vi "Execute_Arc.vi"(2 "Type":u8(slide)=1 min=1 max=12 step=1 scale=1.0..12.0, 3 "Radius":i16 min=0, 4 "occurrence":refnum<k4>, 5 "Motor GPIB":u8=6) -> ()   [LabVIEW 2012]
uses:
  X-Y Go(Global).vi
  <vilib>/express/express arith-compare/Formula/XNode/ExpressFormulaBlockNode.xnode
panel:
  out "move x":i16
  out "move y":i16
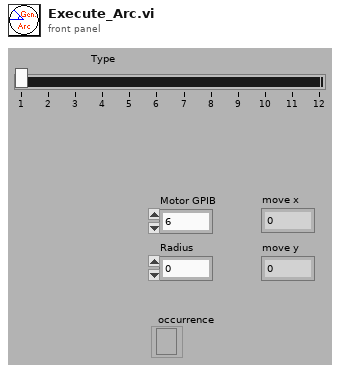
[diagram p1: front panel]
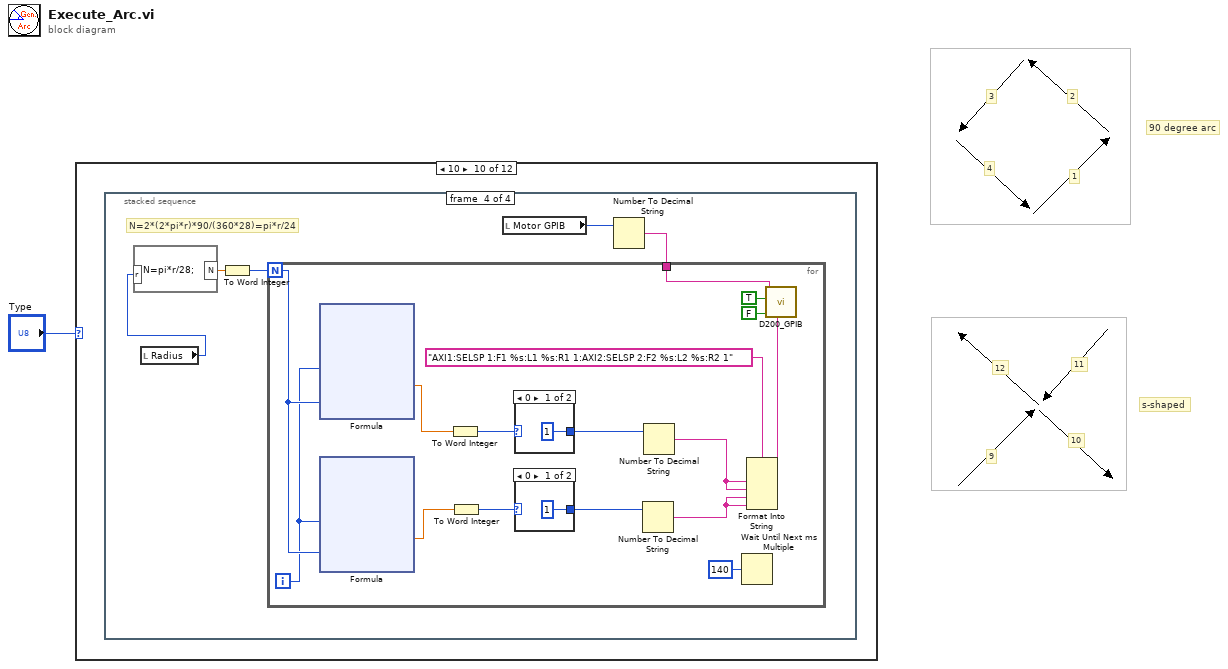
[diagram p0: block diagram]
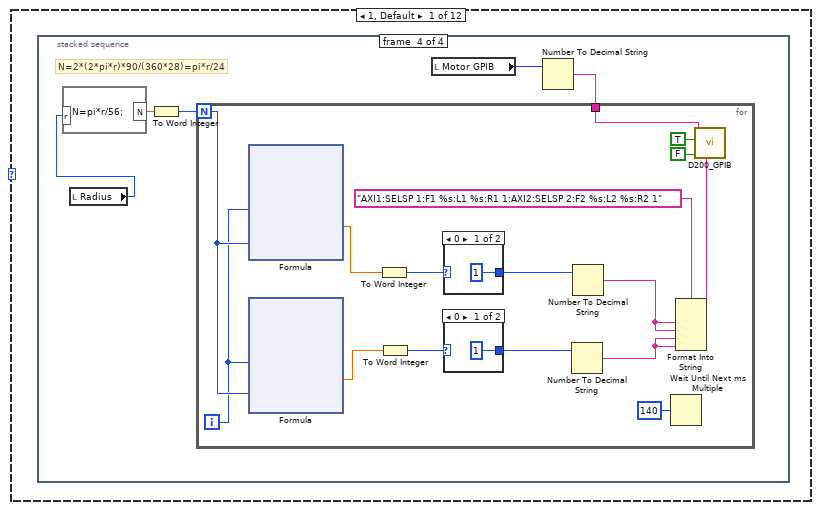
[diagram p2: hidden frame]
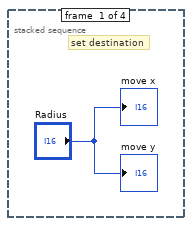
[diagram p3: hidden frame]
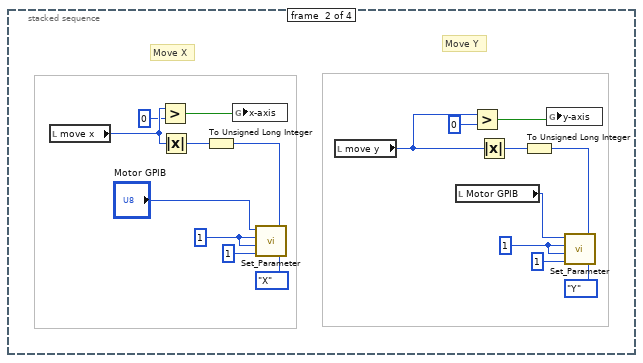
[diagram p4: hidden frame]
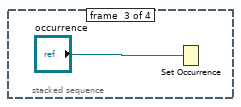
[diagram p5: hidden frame]
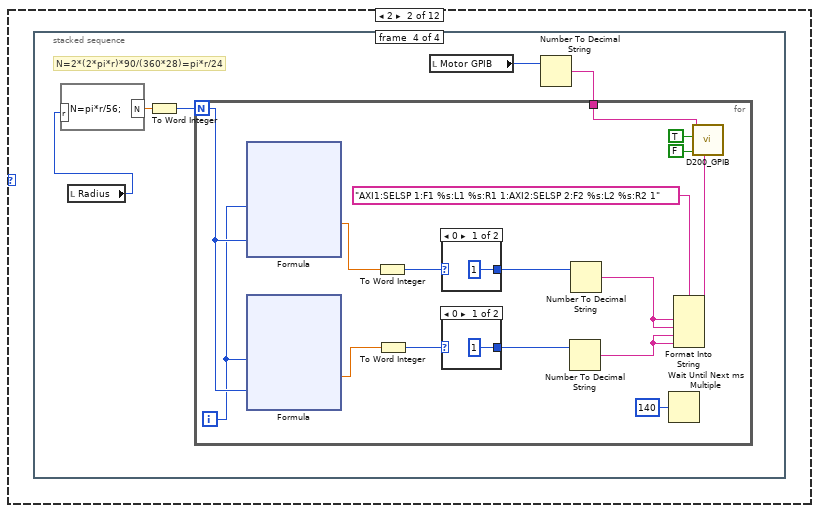
[diagram p8: hidden frame]
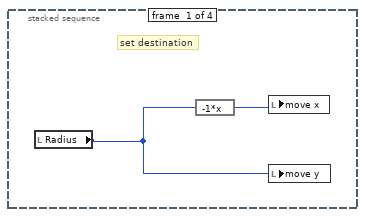
[diagram p9: hidden frame]
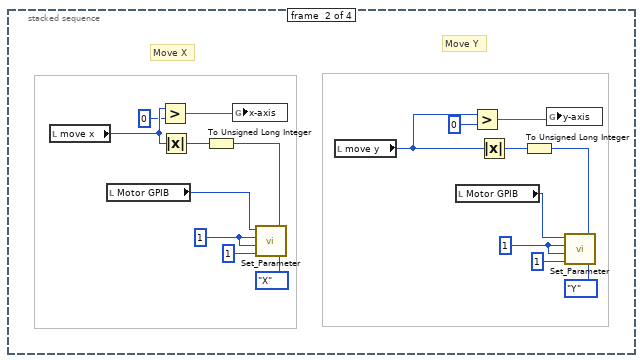
[diagram p10: hidden frame]
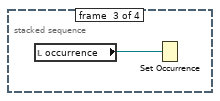
[diagram p11: hidden frame]
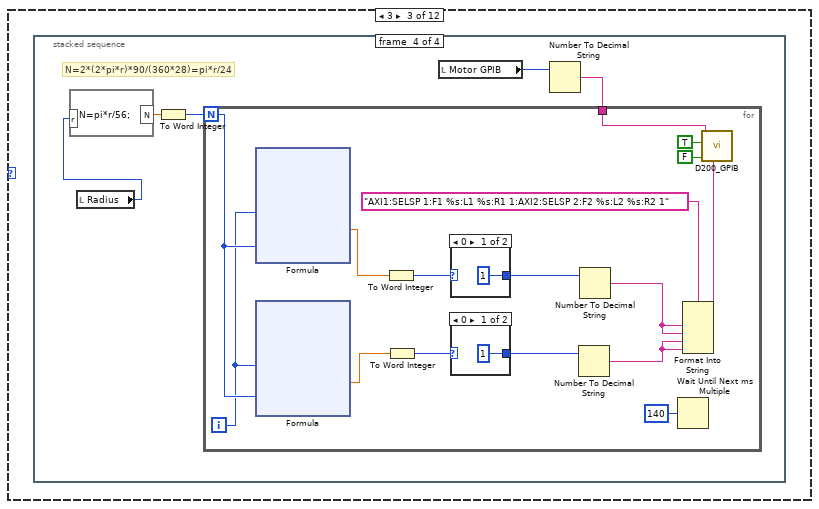
[diagram p14: hidden frame]
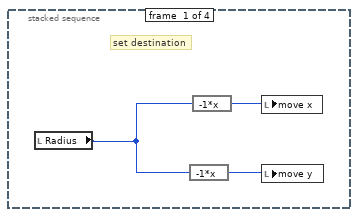
[diagram p15: hidden frame]
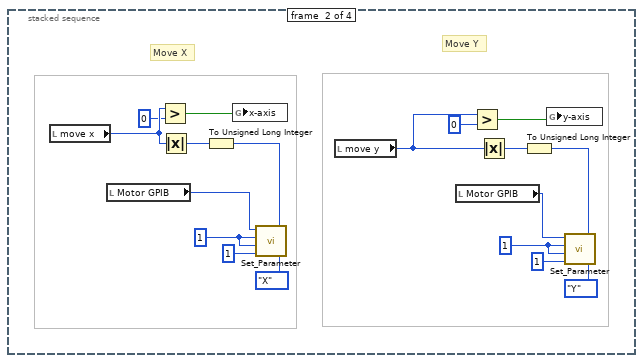
[diagram p16: hidden frame]
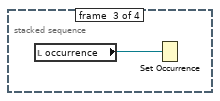
[diagram p17: hidden frame]
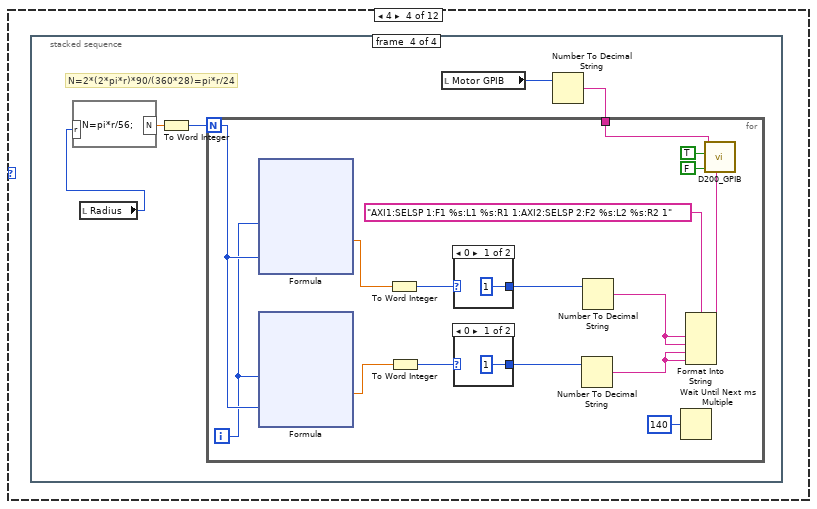
[diagram p20: hidden frame]
diagram:
  # "90 degree arc"
  # "4"
  # "3"
  # "2"
  # "1"
  # "s-shaped"
  # "12"
  # "11"
  # "10"
  # "9"
  n1 = case shown="10" "Type" {
    frame 1, Default {
      n2 = stacked-sequence {
        frame #0 {
          # "set destination"
          "move x" <- "Radius"
          "move y" <- "Radius"
        }
        frame #1 {
          w20 = u16 1 ("L Speed")
          w11 = u16 1 ("L Speed")
          # "Move Y"
          # "Move X"
          n3 = local read "move x"() -> (w12:i16)
          n4 = Greater?(x=w12, y=0) -> (0:w4:bool)
          n5 = Absolute Value(x=w12) -> (abs(x)=w9:i16)
          n6 = To Unsigned Long Integer(number=w9) -> (unsigned 32bit integer=w10:u32)
          n7 = global write "X-Y Go(Global).vi" "x-axis"(w4) -> ()
          n8 = call "Set_Parameter.vi"("Axis"=enum16{"X", "Y", "Z", "U", "V", "W"}."X", "Distance"=w10, "Rate"=u16 1, "L Speed"=w11, "F Speed"=w11, "GPIB_Addr"="Motor GPIB") -> ()
          n9 = local read "move y"() -> (w18:i16)
          n10 = local read "Motor GPIB"() -> (w15:u8)
          n11 = Greater?(x=w18, y=0) -> (0:w5:bool)
          n12 = Absolute Value(x=w18) -> (abs(x)=w17:i16)
          n13 = To Unsigned Long Integer(number=w17) -> (unsigned 32bit integer=w19:u32)
          n14 = global write "X-Y Go(Global).vi" "y-axis"(w5) -> ()
          n15 = call "Set_Parameter.vi"("Axis"=enum16{"X", "Y", "Z", "U", "V", "W"}."Y", "Distance"=w19, "Rate"=u16 1, "L Speed"=w20, "F Speed"=w20, "GPIB_Addr"=w15) -> ()
        }
        frame #2 {
          n16 = Set Occurrence("occurrence") -> ()
        }
        frame #3 {
          # "N=2*(2*pi*r)*90/(360*28)=pi*r/24"
          n17 = local read "Radius"() -> (w22:i16)
          n18 = formula code="N=pi*r/56;"("r"=w22) -> ("N"=w24:dbl)
          n19 = To Word Integer(number=w24) -> (16bit integer=w23:i16)
          n20 = local read "Motor GPIB"() -> (w26:u8)
          n21 = Number To Decimal String(number=w26) -> (decimal integer string=w25:string)  [unwired: 1 in]
          n22 = for {
            N: w23 -> [w35]
            tunnel: w25 -> [w37]
            i -> [w34]
            n23 = xnode "Formula"("i"=w34, "N"=w35) -> ("Result"=w31:dbl)  [unwired: 1 in, 1 out]
            n24 = xnode "Formula"("i"=w34, "N"=w35) -> ("Result"=w33:dbl)  [unwired: 1 in, 1 out]
            n25 = To Word Integer(number=w31) -> (16bit integer=w30:i16)
            n26 = To Word Integer(number=w33) -> (16bit integer=w28:i16)
            n27 = case shown="0" w30 {
              selector: w30 -> [_ w46]
              tunnel: [i16 1 ("16bit integer") w46] -> w29
              frame 0 {
              }
              frame 1, Default {
              }
            }
            n28 = case shown="0" w28 {
              selector: w28 -> [_ w44]
              tunnel: [i16 1 ("16bit integer") w44] -> w27
              frame 0 {
              }
              frame 1, Default {
              }
            }
            n29 = Number To Decimal String(number=w27) -> (decimal integer string=w32:string)  [unwired: 1 in]
            n30 = Number To Decimal String(number=w29) -> (decimal integer string=w39:string)  [unwired: 1 in]
            n31 = Wait Until Next ms Multiple(millisecond multiple=u32 140) -> ()  [unwired: 1 out]
            n32 = Format Into String(format string="AXI1:SELSP 1:F1 %s:L1 %s:R1 1:AXI2:SELSP 2:F2 %s:L2 %s:R2 1", w39, w39, w32, w32) -> (resulting string=w38:string)  [unwired: 2 in, 1 out]
            n33 = call "D200_GPIB.vi"("GPIB\nAddress"=w37, "Write"=TRUE, "Read"=FALSE, "Characters to Write"=w38) -> ()  [unwired: 1 in, 3 out]
          }
        }
      }
    }
    frame 2 {
      n34 = stacked-sequence {
        frame #0 {
          # "set destination"
          n35 = local read "Radius"() -> (w67:i16)
          n36 = expression code="-1*x"(w67) -> (w68:i16)
          n37 = local write "move x"(w68) -> ()
          n38 = local write "move y"(w67) -> ()
        }
        frame #1 {
          w86 = u16 1 ("L Speed")
          w77 = u16 1 ("L Speed")
          # "Move Y"
          # "Move X"
          n39 = local read "move x"() -> (w78:i16)
          n40 = local read "Motor GPIB"() -> (w71:u8)
          n41 = Greater?(x=w78, y=0) -> (0:w69:bool)
          n42 = Absolute Value(x=w78) -> (abs(x)=w75:i16)
          n43 = To Unsigned Long Integer(number=w75) -> (unsigned 32bit integer=w76:u32)
          n44 = global write "X-Y Go(Global).vi" "x-axis"(w69) -> ()
          n45 = call "Set_Parameter.vi"("Axis"=enum16{"X", "Y", "Z", "U", "V", "W"}."X", "Distance"=w76, "Rate"=u16 1, "L Speed"=w77, "F Speed"=w77, "GPIB_Addr"=w71) -> ()
          n46 = local read "move y"() -> (w84:i16)
          n47 = local read "Motor GPIB"() -> (w81:u8)
          n48 = Greater?(x=w84, y=0) -> (0:w70:bool)
          n49 = Absolute Value(x=w84) -> (abs(x)=w83:i16)
          n50 = To Unsigned Long Integer(number=w83) -> (unsigned 32bit integer=w85:u32)
          n51 = global write "X-Y Go(Global).vi" "y-axis"(w70) -> ()
          n52 = call "Set_Parameter.vi"("Axis"=enum16{"X", "Y", "Z", "U", "V", "W"}."Y", "Distance"=w85, "Rate"=u16 1, "L Speed"=w86, "F Speed"=w86, "GPIB_Addr"=w81) -> ()
        }
        frame #2 {
          n53 = local read "occurrence"() -> (w87:refnum<k4>)
          n54 = Set Occurrence(w87) -> ()
        }
        frame #3 {
          # "N=2*(2*pi*r)*90/(360*28)=pi*r/24"
          n55 = local read "Radius"() -> (w88:i16)
          n56 = formula code="N=pi*r/56;"("r"=w88) -> ("N"=w90:dbl)
          n57 = To Word Integer(number=w90) -> (16bit integer=w89:i16)
          n58 = local read "Motor GPIB"() -> (w92:u8)
          n59 = Number To Decimal String(number=w92) -> (decimal integer string=w91:string)  [unwired: 1 in]
          n60 = for {
            N: w89 -> [w101]
            tunnel: w91 -> [w103]
            i -> [w100]
            n61 = xnode "Formula"("i"=w100, "N"=w101) -> ("Result"=w97:dbl)  [unwired: 1 in, 1 out]
            n62 = xnode "Formula"("i"=w100, "N"=w101) -> ("Result"=w99:dbl)  [unwired: 1 in, 1 out]
            n63 = To Word Integer(number=w97) -> (16bit integer=w96:i16)
            n64 = To Word Integer(number=w99) -> (16bit integer=w94:i16)
            n65 = case shown="0" w96 {
              selector: w96 -> [_ w112]
              tunnel: [i16 1 ("16bit integer") w112] -> w95
              frame 0 {
              }
              frame 1, Default {
              }
            }
            n66 = case shown="0" w94 {
              selector: w94 -> [_ w110]
              tunnel: [i16 1 ("16bit integer") w110] -> w93
              frame 0 {
              }
              frame 1, Default {
              }
            }
            n67 = Number To Decimal String(number=w93) -> (decimal integer string=w98:string)  [unwired: 1 in]
            n68 = Number To Decimal String(number=w95) -> (decimal integer string=w105:string)  [unwired: 1 in]
            n69 = Wait Until Next ms Multiple(millisecond multiple=u32 140) -> ()  [unwired: 1 out]
            n70 = Format Into String(format string="AXI1:SELSP 1:F1 %s:L1 %s:R1 1:AXI2:SELSP 2:F2 %s:L2 %s:R2 1", w105, w105, w98, w98) -> (resulting string=w104:string)  [unwired: 2 in, 1 out]
            n71 = call "D200_GPIB.vi"("GPIB\nAddress"=w103, "Write"=TRUE, "Read"=FALSE, "Characters to Write"=w104) -> ()  [unwired: 1 in, 3 out]
          }
        }
      }
    }
    frame 3 {
      n72 = stacked-sequence {
        frame #0 {
          # "set destination"
          n73 = local read "Radius"() -> (w133:i16)
          n74 = expression code="-1*x"(w133) -> (w135:i16)
          n75 = expression code="-1*x"(w133) -> (w134:i16)
          n76 = local write "move x"(w134) -> ()
          n77 = local write "move y"(w135) -> ()
        }
        frame #1 {
          w153 = u16 1 ("L Speed")
          w144 = u16 1 ("L Speed")
          # "Move Y"
          # "Move X"
          n78 = local read "move x"() -> (w145:i16)
          n79 = local read "Motor GPIB"() -> (w138:u8)
          n80 = Greater?(x=w145, y=0) -> (0:w136:bool)
          n81 = Absolute Value(x=w145) -> (abs(x)=w142:i16)
          n82 = To Unsigned Long Integer(number=w142) -> (unsigned 32bit integer=w143:u32)
          n83 = global write "X-Y Go(Global).vi" "x-axis"(w136) -> ()
          n84 = call "Set_Parameter.vi"("Axis"=enum16{"X", "Y", "Z", "U", "V", "W"}."X", "Distance"=w143, "Rate"=u16 1, "L Speed"=w144, "F Speed"=w144, "GPIB_Addr"=w138) -> ()
          n85 = local read "move y"() -> (w151:i16)
          n86 = local read "Motor GPIB"() -> (w148:u8)
          n87 = Greater?(x=w151, y=0) -> (0:w137:bool)
          n88 = Absolute Value(x=w151) -> (abs(x)=w150:i16)
          n89 = To Unsigned Long Integer(number=w150) -> (unsigned 32bit integer=w152:u32)
          n90 = global write "X-Y Go(Global).vi" "y-axis"(w137) -> ()
          n91 = call "Set_Parameter.vi"("Axis"=enum16{"X", "Y", "Z", "U", "V", "W"}."Y", "Distance"=w152, "Rate"=u16 1, "L Speed"=w153, "F Speed"=w153, "GPIB_Addr"=w148) -> ()
        }
        frame #2 {
          n92 = local read "occurrence"() -> (w154:refnum<k4>)
          n93 = Set Occurrence(w154) -> ()
        }
        frame #3 {
          # "N=2*(2*pi*r)*90/(360*28)=pi*r/24"
          n94 = local read "Radius"() -> (w155:i16)
          n95 = formula code="N=pi*r/56;"("r"=w155) -> ("N"=w157:dbl)
          n96 = To Word Integer(number=w157) -> (16bit integer=w156:i16)
          n97 = local read "Motor GPIB"() -> (w159:u8)
          n98 = Number To Decimal String(number=w159) -> (decimal integer string=w158:string)  [unwired: 1 in]
          n99 = for {
            N: w156 -> [w168]
            tunnel: w158 -> [w170]
            i -> [w167]
            n100 = xnode "Formula"("i"=w167, "N"=w168) -> ("Result"=w164:dbl)  [unwired: 1 in, 1 out]
            n101 = xnode "Formula"("i"=w167, "N"=w168) -> ("Result"=w166:dbl)  [unwired: 1 in, 1 out]
            n102 = To Word Integer(number=w164) -> (16bit integer=w163:i16)
            n103 = To Word Integer(number=w166) -> (16bit integer=w161:i16)
            n104 = case shown="0" w163 {
              selector: w163 -> [_ w179]
              tunnel: [i16 1 ("16bit integer") w179] -> w162
              frame 0 {
              }
              frame 1, Default {
              }
            }
            n105 = case shown="0" w161 {
              selector: w161 -> [_ w177]
              tunnel: [i16 1 ("16bit integer") w177] -> w160
              frame 0 {
              }
              frame 1, Default {
              }
            }
            n106 = Number To Decimal String(number=w160) -> (decimal integer string=w165:string)  [unwired: 1 in]
            n107 = Number To Decimal String(number=w162) -> (decimal integer string=w172:string)  [unwired: 1 in]
            n108 = Wait Until Next ms Multiple(millisecond multiple=u32 140) -> ()  [unwired: 1 out]
            n109 = Format Into String(format string="AXI1:SELSP 1:F1 %s:L1 %s:R1 1:AXI2:SELSP 2:F2 %s:L2 %s:R2 1", w172, w172, w165, w165) -> (resulting string=w171:string)  [unwired: 2 in, 1 out]
            n110 = call "D200_GPIB.vi"("GPIB\nAddress"=w170, "Write"=TRUE, "Read"=FALSE, "Characters to Write"=w171) -> ()  [unwired: 1 in, 3 out]
          }
        }
      }
    }
    frame 4 {
      n111 = stacked-sequence {
        frame #0 {
          # "set destination"
          n112 = local read "Radius"() -> (w200:i16)
          n113 = expression code="-1*x"(w200) -> (w201:i16)
          n114 = local write "move x"(w200) -> ()
          n115 = local write "move y"(w201) -> ()
        }
        frame #1 {
          w219 = u16 1 ("L Speed")
          w210 = u16 1 ("L Speed")
          # "Move Y"
          # "Move X"
          n116 = local read "move x"() -> (w211:i16)
          n117 = local read "Motor GPIB"() -> (w204:u8)
          n118 = Greater?(x=w211, y=0) -> (0:w202:bool)
          n119 = Absolute Value(x=w211) -> (abs(x)=w208:i16)
          n120 = To Unsigned Long Integer(number=w208) -> (unsigned 32bit integer=w209:u32)
          n121 = global write "X-Y Go(Global).vi" "x-axis"(w202) -> ()
          n122 = call "Set_Parameter.vi"("Axis"=enum16{"X", "Y", "Z", "U", "V", "W"}."X", "Distance"=w209, "Rate"=u16 1, "L Speed"=w210, "F Speed"=w210, "GPIB_Addr"=w204) -> ()
          n123 = local read "move y"() -> (w217:i16)
          n124 = local read "Motor GPIB"() -> (w214:u8)
          n125 = Greater?(x=w217, y=0) -> (0:w203:bool)
          n126 = Absolute Value(x=w217) -> (abs(x)=w216:i16)
          n127 = To Unsigned Long Integer(number=w216) -> (unsigned 32bit integer=w218:u32)
          n128 = global write "X-Y Go(Global).vi" "y-axis"(w203) -> ()
          n129 = call "Set_Parameter.vi"("Axis"=enum16{"X", "Y", "Z", "U", "V", "W"}."Y", "Distance"=w218, "Rate"=u16 1, "L Speed"=w219, "F Speed"=w219, "GPIB_Addr"=w214) -> ()
        }
        frame #2 {
          n130 = local read "occurrence"() -> (w220:refnum<k4>)
          n131 = Set Occurrence(w220) -> ()
        }
        frame #3 {
          # "N=2*(2*pi*r)*90/(360*28)=pi*r/24"
          n132 = local read "Radius"() -> (w221:i16)
          n133 = formula code="N=pi*r/56;"("r"=w221) -> ("N"=w223:dbl)
          n134 = To Word Integer(number=w223) -> (16bit integer=w222:i16)
          n135 = local read "Motor GPIB"() -> (w225:u8)
          n136 = Number To Decimal String(number=w225) -> (decimal integer string=w224:string)  [unwired: 1 in]
          n137 = for {
            N: w222 -> [w234]
            tunnel: w224 -> [w236]
            i -> [w233]
            n138 = xnode "Formula"("i"=w233, "N"=w234) -> ("Result"=w230:dbl)  [unwired: 1 in, 1 out]
            n139 = xnode "Formula"("i"=w233, "N"=w234) -> ("Result"=w232:dbl)  [unwired: 1 in, 1 out]
            n140 = To Word Integer(number=w230) -> (16bit integer=w229:i16)
            n141 = To Word Integer(number=w232) -> (16bit integer=w227:i16)
            n142 = case shown="0" w229 {
              selector: w229 -> [_ w245]
              tunnel: [i16 1 ("16bit integer") w245] -> w228
              frame 0 {
              }
              frame 1, Default {
              }
            }
            n143 = case shown="0" w227 {
              selector: w227 -> [_ w243]
              tunnel: [i16 1 ("16bit integer") w243] -> w226
              frame 0 {
              }
              frame 1, Default {
              }
            }
            n144 = Number To Decimal String(number=w226) -> (decimal integer string=w231:string)  [unwired: 1 in]
            n145 = Number To Decimal String(number=w228) -> (decimal integer string=w238:string)  [unwired: 1 in]
            n146 = Wait Until Next ms Multiple(millisecond multiple=u32 140) -> ()  [unwired: 1 out]
            n147 = Format Into String(format string="AXI1:SELSP 1:F1 %s:L1 %s:R1 1:AXI2:SELSP 2:F2 %s:L2 %s:R2 1", w238, w238, w231, w231) -> (resulting string=w237:string)  [unwired: 2 in, 1 out]
            n148 = call "D200_GPIB.vi"("GPIB\nAddress"=w236, "Write"=TRUE, "Read"=FALSE, "Characters to Write"=w237) -> ()  [unwired: 1 in, 3 out]
          }
        }
      }
    }
    frame 5 {
      n149 = stacked-sequence {
        frame #0 {
          n150 = local read "Radius"() -> (w266:i16)
          n151 = local write "move x"(w266) -> ()
          n152 = local write "move y"(w266) -> ()
        }
        frame #1 {
          w284 = u16 1 ("L Speed")
          w275 = u16 1 ("L Speed")
          # "Move Y"
          # "Move X"
          n153 = local read "move x"() -> (w276:i16)
          n154 = local read "Motor GPIB"() -> (w269:u8)
          n155 = Greater?(x=w276, y=0) -> (0:w267:bool)
          n156 = Absolute Value(x=w276) -> (abs(x)=w273:i16)
          n157 = To Unsigned Long Integer(number=w273) -> (unsigned 32bit integer=w274:u32)
          n158 = global write "X-Y Go(Global).vi" "x-axis"(w267) -> ()
          n159 = call "Set_Parameter.vi"("Axis"=enum16{"X", "Y", "Z", "U", "V", "W"}."X", "Distance"=w274, "Rate"=u16 1, "L Speed"=w275, "F Speed"=w275, "GPIB_Addr"=w269) -> ()
          n160 = local read "move y"() -> (w282:i16)
          n161 = local read "Motor GPIB"() -> (w279:u8)
          n162 = Greater?(x=w282, y=0) -> (0:w268:bool)
          n163 = Absolute Value(x=w282) -> (abs(x)=w281:i16)
          n164 = To Unsigned Long Integer(number=w281) -> (unsigned 32bit integer=w283:u32)
          n165 = global write "X-Y Go(Global).vi" "y-axis"(w268) -> ()
          n166 = call "Set_Parameter.vi"("Axis"=enum16{"X", "Y", "Z", "U", "V", "W"}."Y", "Distance"=w283, "Rate"=u16 1, "L Speed"=w284, "F Speed"=w284, "GPIB_Addr"=w279) -> ()
        }
        frame #2 {
          # "N=2*(2*pi*r)*90/(360*28)=pi*r/24"
          n167 = local read "Radius"() -> (w285:i16)
          n168 = formula code="N=pi*r/56;"("r"=w285) -> ("N"=w287:dbl)
          n169 = To Word Integer(number=w287) -> (16bit integer=w286:i16)
          n170 = local read "Motor GPIB"() -> (w289:u8)
          n171 = Number To Decimal String(number=w289) -> (decimal integer string=w288:string)  [unwired: 1 in]
          n172 = for {
            N: w286 -> [w298]
            tunnel: w288 -> [w300]
            i -> [w297]
            n173 = xnode "Formula"("i"=w297, "N"=w298) -> ("Result"=w294:dbl)  [unwired: 1 in, 1 out]
            n174 = xnode "Formula"("i"=w297, "N"=w298) -> ("Result"=w296:dbl)  [unwired: 1 in, 1 out]
            n175 = To Word Integer(number=w294) -> (16bit integer=w293:i16)
            n176 = To Word Integer(number=w296) -> (16bit integer=w291:i16)
            n177 = case shown="0" w293 {
              selector: w293 -> [_ w309]
              tunnel: [i16 1 ("16bit integer") w309] -> w292
              frame 0 {
              }
              frame 1, Default {
              }
            }
            n178 = case shown="0" w291 {
              selector: w291 -> [_ w307]
              tunnel: [i16 1 ("16bit integer") w307] -> w290
              frame 0 {
              }
              frame 1, Default {
              }
            }
            n179 = Number To Decimal String(number=w290) -> (decimal integer string=w295:string)  [unwired: 1 in]
            n180 = Number To Decimal String(number=w292) -> (decimal integer string=w302:string)  [unwired: 1 in]
            n181 = Wait Until Next ms Multiple(millisecond multiple=u32 140) -> ()  [unwired: 1 out]
            n182 = Format Into String(format string="AXI1:SELSP 1:F1 %s:L1 %s:R1 1:AXI2:SELSP 2:F2 %s:L2 %s:R2 1", w302, w302, w295, w295) -> (resulting string=w301:string)  [unwired: 2 in, 1 out]
            n183 = call "D200_GPIB.vi"("GPIB\nAddress"=w300, "Write"=TRUE, "Read"=FALSE, "Characters to Write"=w301) -> ()  [unwired: 1 in, 3 out]
          }
        }
      }
    }
    frame 6 {
      n184 = stacked-sequence {
        frame #0 {
          n185 = local read "Radius"() -> (w331:i16)
          n186 = expression code="x*(-1)"(w331) -> (w330:i16)
          n187 = local write "move x"(w331) -> ()
          n188 = local write "move y"(w330) -> ()
        }
        frame #1 {
          w349 = u16 1 ("L Speed")
          w340 = u16 1 ("L Speed")
          # "Move Y"
          # "Move X"
          n189 = local read "move x"() -> (w341:i16)
          n190 = local read "Motor GPIB"() -> (w334:u8)
          n191 = Greater?(x=w341, y=0) -> (0:w332:bool)
          n192 = Absolute Value(x=w341) -> (abs(x)=w338:i16)
          n193 = To Unsigned Long Integer(number=w338) -> (unsigned 32bit integer=w339:u32)
          n194 = global write "X-Y Go(Global).vi" "x-axis"(w332) -> ()
          n195 = call "Set_Parameter.vi"("Axis"=enum16{"X", "Y", "Z", "U", "V", "W"}."X", "Distance"=w339, "Rate"=u16 1, "L Speed"=w340, "F Speed"=w340, "GPIB_Addr"=w334) -> ()
          n196 = local read "move y"() -> (w347:i16)
          n197 = local read "Motor GPIB"() -> (w344:u8)
          n198 = Greater?(x=w347, y=0) -> (0:w333:bool)
          n199 = Absolute Value(x=w347) -> (abs(x)=w346:i16)
          n200 = To Unsigned Long Integer(number=w346) -> (unsigned 32bit integer=w348:u32)
          n201 = global write "X-Y Go(Global).vi" "y-axis"(w333) -> ()
          n202 = call "Set_Parameter.vi"("Axis"=enum16{"X", "Y", "Z", "U", "V", "W"}."Y", "Distance"=w348, "Rate"=u16 1, "L Speed"=w349, "F Speed"=w349, "GPIB_Addr"=w344) -> ()
        }
        frame #2 {
          # "N=2*(2*pi*r)*90/(360*28)=pi*r/24"
          n203 = local read "Radius"() -> (w350:i16)
          n204 = formula code="N=pi*r/56;"("r"=w350) -> ("N"=w352:dbl)
          n205 = To Word Integer(number=w352) -> (16bit integer=w351:i16)
          n206 = local read "Motor GPIB"() -> (w354:u8)
          n207 = Number To Decimal String(number=w354) -> (decimal integer string=w353:string)  [unwired: 1 in]
          n208 = for {
            N: w351 -> [w363]
            tunnel: w353 -> [w365]
            i -> [w362]
            n209 = xnode "Formula"("i"=w362, "N"=w363) -> ("Result"=w359:dbl)  [unwired: 1 in, 1 out]
            n210 = xnode "Formula"("i"=w362, "N"=w363) -> ("Result"=w361:dbl)  [unwired: 1 in, 1 out]
            n211 = To Word Integer(number=w359) -> (16bit integer=w358:i16)
            n212 = To Word Integer(number=w361) -> (16bit integer=w356:i16)
            n213 = case shown="0" w358 {
              selector: w358 -> [_ w374]
              tunnel: [i16 1 ("16bit integer") w374] -> w357
              frame 0 {
              }
              frame 1, Default {
              }
            }
            n214 = case shown="0" w356 {
              selector: w356 -> [_ w372]
              tunnel: [i16 1 ("16bit integer") w372] -> w355
              frame 0 {
              }
              frame 1, Default {
              }
            }
            n215 = Number To Decimal String(number=w355) -> (decimal integer string=w360:string)  [unwired: 1 in]
            n216 = Number To Decimal String(number=w357) -> (decimal integer string=w367:string)  [unwired: 1 in]
            n217 = Wait Until Next ms Multiple(millisecond multiple=u32 140) -> ()  [unwired: 1 out]
            n218 = Format Into String(format string="AXI1:SELSP 1:F1 %s:L1 %s:R1 1:AXI2:SELSP 2:F2 %s:L2 %s:R2 1", w367, w367, w360, w360) -> (resulting string=w366:string)  [unwired: 2 in, 1 out]
            n219 = call "D200_GPIB.vi"("GPIB\nAddress"=w365, "Write"=TRUE, "Read"=FALSE, "Characters to Write"=w366) -> ()  [unwired: 1 in, 3 out]
          }
        }
      }
    }
    frame 7 {
      n220 = stacked-sequence {
        frame #0 {
          n221 = local read "Radius"() -> (w397:i16)
          n222 = expression code="x*(-1)"(w397) -> (w395:i16)
          n223 = expression code="x*(-1)"(w397) -> (w396:i16)
          n224 = local write "move x"(w395) -> ()
          n225 = local write "move y"(w396) -> ()
        }
        frame #1 {
          w415 = u16 1 ("L Speed")
          w406 = u16 1 ("L Speed")
          # "Move Y"
          # "Move X"
          n226 = local read "move x"() -> (w407:i16)
          n227 = local read "Motor GPIB"() -> (w400:u8)
          n228 = Greater?(x=w407, y=0) -> (0:w398:bool)
          n229 = Absolute Value(x=w407) -> (abs(x)=w404:i16)
          n230 = To Unsigned Long Integer(number=w404) -> (unsigned 32bit integer=w405:u32)
          n231 = global write "X-Y Go(Global).vi" "x-axis"(w398) -> ()
          n232 = call "Set_Parameter.vi"("Axis"=enum16{"X", "Y", "Z", "U", "V", "W"}."X", "Distance"=w405, "Rate"=u16 1, "L Speed"=w406, "F Speed"=w406, "GPIB_Addr"=w400) -> ()
          n233 = local read "move y"() -> (w413:i16)
          n234 = local read "Motor GPIB"() -> (w410:u8)
          n235 = Greater?(x=w413, y=0) -> (0:w399:bool)
          n236 = Absolute Value(x=w413) -> (abs(x)=w412:i16)
          n237 = To Unsigned Long Integer(number=w412) -> (unsigned 32bit integer=w414:u32)
          n238 = global write "X-Y Go(Global).vi" "y-axis"(w399) -> ()
          n239 = call "Set_Parameter.vi"("Axis"=enum16{"X", "Y", "Z", "U", "V", "W"}."Y", "Distance"=w414, "Rate"=u16 1, "L Speed"=w415, "F Speed"=w415, "GPIB_Addr"=w410) -> ()
        }
        frame #2 {
          # "N=2*(2*pi*r)*90/(360*28)=pi*r/24"
          n240 = local read "Radius"() -> (w416:i16)
          n241 = formula code="N=pi*r/56;"("r"=w416) -> ("N"=w418:dbl)
          n242 = To Word Integer(number=w418) -> (16bit integer=w417:i16)
          n243 = local read "Motor GPIB"() -> (w420:u8)
          n244 = Number To Decimal String(number=w420) -> (decimal integer string=w419:string)  [unwired: 1 in]
          n245 = for {
            N: w417 -> [w429]
            tunnel: w419 -> [w431]
            i -> [w428]
            n246 = xnode "Formula"("i"=w428, "N"=w429) -> ("Result"=w425:dbl)  [unwired: 1 in, 1 out]
            n247 = xnode "Formula"("i"=w428, "N"=w429) -> ("Result"=w427:dbl)  [unwired: 1 in, 1 out]
            n248 = To Word Integer(number=w425) -> (16bit integer=w424:i16)
            n249 = To Word Integer(number=w427) -> (16bit integer=w422:i16)
            n250 = case shown="0" w424 {
              selector: w424 -> [_ w440]
              tunnel: [i16 1 ("16bit integer") w440] -> w423
              frame 0 {
              }
              frame 1, Default {
              }
            }
            n251 = case shown="0" w422 {
              selector: w422 -> [_ w438]
              tunnel: [i16 1 ("16bit integer") w438] -> w421
              frame 0 {
              }
              frame 1, Default {
              }
            }
            n252 = Number To Decimal String(number=w421) -> (decimal integer string=w426:string)  [unwired: 1 in]
            n253 = Number To Decimal String(number=w423) -> (decimal integer string=w433:string)  [unwired: 1 in]
            n254 = Wait Until Next ms Multiple(millisecond multiple=u32 140) -> ()  [unwired: 1 out]
            n255 = Format Into String(format string="AXI1:SELSP 1:F1 %s:L1 %s:R1 1:AXI2:SELSP 2:F2 %s:L2 %s:R2 1", w433, w433, w426, w426) -> (resulting string=w432:string)  [unwired: 2 in, 1 out]
            n256 = call "D200_GPIB.vi"("GPIB\nAddress"=w431, "Write"=TRUE, "Read"=FALSE, "Characters to Write"=w432) -> ()  [unwired: 1 in, 3 out]
          }
        }
      }
    }
    frame 8 {
      n257 = stacked-sequence {
        frame #0 {
          n258 = local read "Radius"() -> (w462:i16)
          n259 = expression code="x*(-1)"(w462) -> (w461:i16)
          n260 = local write "move x"(w461) -> ()
          n261 = local write "move y"(w462) -> ()
        }
        frame #1 {
          w480 = u16 1 ("L Speed")
          w471 = u16 1 ("L Speed")
          # "Move Y"
          # "Move X"
          n262 = local read "move x"() -> (w472:i16)
          n263 = local read "Motor GPIB"() -> (w465:u8)
          n264 = Greater?(x=w472, y=0) -> (0:w463:bool)
          n265 = Absolute Value(x=w472) -> (abs(x)=w469:i16)
          n266 = To Unsigned Long Integer(number=w469) -> (unsigned 32bit integer=w470:u32)
          n267 = global write "X-Y Go(Global).vi" "x-axis"(w463) -> ()
          n268 = call "Set_Parameter.vi"("Axis"=enum16{"X", "Y", "Z", "U", "V", "W"}."X", "Distance"=w470, "Rate"=u16 1, "L Speed"=w471, "F Speed"=w471, "GPIB_Addr"=w465) -> ()
          n269 = local read "move y"() -> (w478:i16)
          n270 = local read "Motor GPIB"() -> (w475:u8)
          n271 = Greater?(x=w478, y=0) -> (0:w464:bool)
          n272 = Absolute Value(x=w478) -> (abs(x)=w477:i16)
          n273 = To Unsigned Long Integer(number=w477) -> (unsigned 32bit integer=w479:u32)
          n274 = global write "X-Y Go(Global).vi" "y-axis"(w464) -> ()
          n275 = call "Set_Parameter.vi"("Axis"=enum16{"X", "Y", "Z", "U", "V", "W"}."Y", "Distance"=w479, "Rate"=u16 1, "L Speed"=w480, "F Speed"=w480, "GPIB_Addr"=w475) -> ()
        }
        frame #2 {
          # "N=2*(2*pi*r)*90/(360*28)=pi*r/24"
          n276 = local read "Radius"() -> (w481:i16)
          n277 = formula code="N=pi*r/56;"("r"=w481) -> ("N"=w483:dbl)
          n278 = To Word Integer(number=w483) -> (16bit integer=w482:i16)
          n279 = local read "Motor GPIB"() -> (w485:u8)
          n280 = Number To Decimal String(number=w485) -> (decimal integer string=w484:string)  [unwired: 1 in]
          n281 = for {
            N: w482 -> [w494]
            tunnel: w484 -> [w496]
            i -> [w493]
            n282 = xnode "Formula"("i"=w493, "N"=w494) -> ("Result"=w490:dbl)  [unwired: 1 in, 1 out]
            n283 = xnode "Formula"("i"=w493, "N"=w494) -> ("Result"=w492:dbl)  [unwired: 1 in, 1 out]
            n284 = To Word Integer(number=w490) -> (16bit integer=w489:i16)
            n285 = To Word Integer(number=w492) -> (16bit integer=w487:i16)
            n286 = case shown="0" w489 {
              selector: w489 -> [_ w505]
              tunnel: [i16 1 ("16bit integer") w505] -> w488
              frame 0 {
              }
              frame 1, Default {
              }
            }
            n287 = case shown="0" w487 {
              selector: w487 -> [_ w503]
              tunnel: [i16 1 ("16bit integer") w503] -> w486
              frame 0 {
              }
              frame 1, Default {
              }
            }
            n288 = Number To Decimal String(number=w486) -> (decimal integer string=w491:string)  [unwired: 1 in]
            n289 = Number To Decimal String(number=w488) -> (decimal integer string=w498:string)  [unwired: 1 in]
            n290 = Wait Until Next ms Multiple(millisecond multiple=u32 140) -> ()  [unwired: 1 out]
            n291 = Format Into String(format string="AXI1:SELSP 1:F1 %s:L1 %s:R1 1:AXI2:SELSP 2:F2 %s:L2 %s:R2 1", w498, w498, w491, w491) -> (resulting string=w497:string)  [unwired: 2 in, 1 out]
            n292 = call "D200_GPIB.vi"("GPIB\nAddress"=w496, "Write"=TRUE, "Read"=FALSE, "Characters to Write"=w497) -> ()  [unwired: 1 in, 3 out]
          }
        }
      }
    }
    frame 9 {
      n293 = stacked-sequence {
        frame #0 {
          n294 = local read "Radius"() -> (w527:i16)
          n295 = expression code="2*x"(w527) -> (w526:i16)
          n296 = local write "move x"(w526) -> ()
          n297 = local write "move y"(w526) -> ()
        }
        frame #1 {
          w545 = u16 1 ("L Speed")
          w536 = u16 1 ("L Speed")
          # "Move Y"
          # "Move X"
          n298 = local read "move x"() -> (w537:i16)
          n299 = local read "Motor GPIB"() -> (w530:u8)
          n300 = Greater?(x=w537, y=0) -> (0:w528:bool)
          n301 = Absolute Value(x=w537) -> (abs(x)=w534:i16)
          n302 = To Unsigned Long Integer(number=w534) -> (unsigned 32bit integer=w535:u32)
          n303 = global write "X-Y Go(Global).vi" "x-axis"(w528) -> ()
          n304 = call "Set_Parameter.vi"("Axis"=enum16{"X", "Y", "Z", "U", "V", "W"}."X", "Distance"=w535, "Rate"=u16 1, "L Speed"=w536, "F Speed"=w536, "GPIB_Addr"=w530) -> ()
          n305 = local read "move y"() -> (w543:i16)
          n306 = local read "Motor GPIB"() -> (w540:u8)
          n307 = Greater?(x=w543, y=0) -> (0:w529:bool)
          n308 = Absolute Value(x=w543) -> (abs(x)=w542:i16)
          n309 = To Unsigned Long Integer(number=w542) -> (unsigned 32bit integer=w544:u32)
          n310 = global write "X-Y Go(Global).vi" "y-axis"(w529) -> ()
          n311 = call "Set_Parameter.vi"("Axis"=enum16{"X", "Y", "Z", "U", "V", "W"}."Y", "Distance"=w544, "Rate"=u16 1, "L Speed"=w545, "F Speed"=w545, "GPIB_Addr"=w540) -> ()
        }
        frame #2 {
          n312 = local read "occurrence"() -> (w546:refnum<k4>)
          n313 = Set Occurrence(w546) -> ()
        }
        frame #3 {
          # "N=2*(2*pi*r)*90/(360*28)=pi*r/24"
          n314 = local read "Radius"() -> (w547:i16)
          n315 = formula code="N=pi*r/28;"("r"=w547) -> ("N"=w549:dbl)
          n316 = To Word Integer(number=w549) -> (16bit integer=w548:i16)
          n317 = local read "Motor GPIB"() -> (w551:u8)
          n318 = Number To Decimal String(number=w551) -> (decimal integer string=w550:string)  [unwired: 1 in]
          n319 = for {
            N: w548 -> [w560]
            tunnel: w550 -> [w562]
            i -> [w559]
            n320 = xnode "Formula"("i"=w559, "N"=w560) -> ("Result"=w556:dbl)  [unwired: 1 in, 1 out]
            n321 = xnode "Formula"("i"=w559, "N"=w560) -> ("Result"=w558:dbl)  [unwired: 1 in, 1 out]
            n322 = To Word Integer(number=w556) -> (16bit integer=w555:i16)
            n323 = To Word Integer(number=w558) -> (16bit integer=w553:i16)
            n324 = case shown="0" w555 {
              selector: w555 -> [_ w571]
              tunnel: [i16 1 ("16bit integer") w571] -> w554
              frame 0 {
              }
              frame 1, Default {
              }
            }
            n325 = case shown="0" w553 {
              selector: w553 -> [_ w569]
              tunnel: [i16 1 ("16bit integer") w569] -> w552
              frame 0 {
              }
              frame 1, Default {
              }
            }
            n326 = Number To Decimal String(number=w552) -> (decimal integer string=w557:string)  [unwired: 1 in]
            n327 = Number To Decimal String(number=w554) -> (decimal integer string=w564:string)  [unwired: 1 in]
            n328 = Wait Until Next ms Multiple(millisecond multiple=u32 140) -> ()  [unwired: 1 out]
            n329 = Format Into String(format string="AXI1:SELSP 1:F1 %s:L1 %s:R1 1:AXI2:SELSP 2:F2 %s:L2 %s:R2 1", w564, w564, w557, w557) -> (resulting string=w563:string)  [unwired: 2 in, 1 out]
            n330 = call "D200_GPIB.vi"("GPIB\nAddress"=w562, "Write"=TRUE, "Read"=FALSE, "Characters to Write"=w563) -> ()  [unwired: 1 in, 3 out]
          }
        }
      }
    }
    frame 10 {
      n331 = stacked-sequence {
        frame #0 {
          n332 = local read "Radius"() -> (w593:i16)
          n333 = expression code="2*x"(w593) -> (w592:i16)
          n334 = expression code="-2*x"(w593) -> (w594:i16)
          n335 = local write "move x"(w592) -> ()
          n336 = local write "move y"(w594) -> ()
        }
        frame #1 {
          w612 = u16 1 ("L Speed")
          w603 = u16 1 ("L Speed")
          # "Move Y"
          # "Move X"
          n337 = local read "move x"() -> (w604:i16)
          n338 = local read "Motor GPIB"() -> (w597:u8)
          n339 = Greater?(x=w604, y=0) -> (0:w596:bool)
          n340 = Absolute Value(x=w604) -> (abs(x)=w601:i16)
          n341 = global write "X-Y Go(Global).vi" "x-axis"(w596) -> ()
          n342 = To Unsigned Long Integer(number=w601) -> (unsigned 32bit integer=w602:u32)
          n343 = call "Set_Parameter.vi"("Axis"=enum16{"X", "Y", "Z", "U", "V", "W"}."X", "Distance"=w602, "Rate"=u16 1, "L Speed"=w603, "F Speed"=w603, "GPIB_Addr"=w597) -> ()
          n344 = local read "move y"() -> (w610:i16)
          n345 = local read "Motor GPIB"() -> (w607:u8)
          n346 = Greater?(x=w610, y=0) -> (0:w595:bool)
          n347 = Absolute Value(x=w610) -> (abs(x)=w609:i16)
          n348 = global write "X-Y Go(Global).vi" "y-axis"(w595) -> ()
          n349 = To Unsigned Long Integer(number=w609) -> (unsigned 32bit integer=w611:u32)
          n350 = call "Set_Parameter.vi"("Axis"=enum16{"X", "Y", "Z", "U", "V", "W"}."Y", "Distance"=w611, "Rate"=u16 1, "L Speed"=w612, "F Speed"=w612, "GPIB_Addr"=w607) -> ()
        }
        frame #2 {
          n351 = local read "occurrence"() -> (w613:refnum<k4>)
          n352 = Set Occurrence(w613) -> ()
        }
        frame #3 {
          # "N=2*(2*pi*r)*90/(360*28)=pi*r/24"
          n353 = local read "Radius"() -> (w614:i16)
          n354 = formula code="N=pi*r/28;"("r"=w614) -> ("N"=w616:dbl)
          n355 = To Word Integer(number=w616) -> (16bit integer=w615:i16)
          n356 = local read "Motor GPIB"() -> (w618:u8)
          n357 = Number To Decimal String(number=w618) -> (decimal integer string=w617:string)  [unwired: 1 in]
          n358 = for {
            N: w615 -> [w627]
            tunnel: w617 -> [w629]
            i -> [w626]
            n359 = xnode "Formula"("i"=w626, "N"=w627) -> ("Result"=w623:dbl)  [unwired: 1 in, 1 out]
            n360 = xnode "Formula"("i"=w626, "N"=w627) -> ("Result"=w625:dbl)  [unwired: 1 in, 1 out]
            n361 = To Word Integer(number=w623) -> (16bit integer=w622:i16)
            n362 = To Word Integer(number=w625) -> (16bit integer=w620:i16)
            n363 = case shown="0" w622 {
              selector: w622 -> [_ w638]
              tunnel: [i16 1 ("16bit integer") w638] -> w621
              frame 0 {
              }
              frame 1, Default {
              }
            }
            n364 = case shown="0" w620 {
              selector: w620 -> [_ w636]
              tunnel: [i16 1 ("16bit integer") w636] -> w619
              frame 0 {
              }
              frame 1, Default {
              }
            }
            n365 = Number To Decimal String(number=w619) -> (decimal integer string=w624:string)  [unwired: 1 in]
            n366 = Number To Decimal String(number=w621) -> (decimal integer string=w631:string)  [unwired: 1 in]
            n367 = Wait Until Next ms Multiple(millisecond multiple=u32 140) -> ()  [unwired: 1 out]
            n368 = Format Into String(format string="AXI1:SELSP 1:F1 %s:L1 %s:R1 1:AXI2:SELSP 2:F2 %s:L2 %s:R2 1", w631, w631, w624, w624) -> (resulting string=w630:string)  [unwired: 2 in, 1 out]
            n369 = call "D200_GPIB.vi"("GPIB\nAddress"=w629, "Write"=TRUE, "Read"=FALSE, "Characters to Write"=w630) -> ()  [unwired: 1 in, 3 out]
          }
        }
      }
    }
    frame 11 {
      n370 = stacked-sequence {
        frame #0 {
          n371 = local read "Radius"() -> (w660:i16)
          n372 = expression code="-2*x"(w660) -> (w659:i16)
          n373 = expression code="-2*x"(w660) -> (w661:i16)
          n374 = local write "move x"(w659) -> ()
          n375 = local write "move y"(w661) -> ()
        }
        frame #1 {
          w679 = u16 1 ("L Speed")
          w670 = u16 1 ("L Speed")
          # "Move Y"
          # "Move X"
          n376 = local read "move x"() -> (w671:i16)
          n377 = local read "Motor GPIB"() -> (w664:u8)
          n378 = Greater?(x=w671, y=0) -> (0:w663:bool)
          n379 = Absolute Value(x=w671) -> (abs(x)=w668:i16)
          n380 = global write "X-Y Go(Global).vi" "x-axis"(w663) -> ()
          n381 = To Unsigned Long Integer(number=w668) -> (unsigned 32bit integer=w669:u32)
          n382 = call "Set_Parameter.vi"("Axis"=enum16{"X", "Y", "Z", "U", "V", "W"}."X", "Distance"=w669, "Rate"=u16 1, "L Speed"=w670, "F Speed"=w670, "GPIB_Addr"=w664) -> ()
          n383 = local read "move y"() -> (w677:i16)
          n384 = local read "Motor GPIB"() -> (w674:u8)
          n385 = Greater?(x=w677, y=0) -> (0:w662:bool)
          n386 = Absolute Value(x=w677) -> (abs(x)=w676:i16)
          n387 = global write "X-Y Go(Global).vi" "y-axis"(w662) -> ()
          n388 = To Unsigned Long Integer(number=w676) -> (unsigned 32bit integer=w678:u32)
          n389 = call "Set_Parameter.vi"("Axis"=enum16{"X", "Y", "Z", "U", "V", "W"}."Y", "Distance"=w678, "Rate"=u16 1, "L Speed"=w679, "F Speed"=w679, "GPIB_Addr"=w674) -> ()
        }
        frame #2 {
          n390 = local read "occurrence"() -> (w680:refnum<k4>)
          n391 = Set Occurrence(w680) -> ()
        }
        frame #3 {
          # "N=2*(2*pi*r)*90/(360*28)=pi*r/24"
          n392 = local read "Radius"() -> (w685:i16)
          n393 = formula code="N=pi*r/28;"("r"=w685) -> ("N"=w683:dbl)
          n394 = To Word Integer(number=w683) -> (16bit integer=w684:i16)
          n395 = local read "Motor GPIB"() -> (w681:u8)
          n396 = Number To Decimal String(number=w681) -> (decimal integer string=w682:string)  [unwired: 1 in]
          n397 = for {
            N: w684 -> [w694]
            tunnel: w682 -> [w696]
            i -> [w693]
            n398 = xnode "Formula"("i"=w693, "N"=w694) -> ("Result"=w690:dbl)  [unwired: 1 in, 1 out]
            n399 = xnode "Formula"("i"=w693, "N"=w694) -> ("Result"=w692:dbl)  [unwired: 1 in, 1 out]
            n400 = To Word Integer(number=w690) -> (16bit integer=w689:i16)
            n401 = To Word Integer(number=w692) -> (16bit integer=w687:i16)
            n402 = case shown="0" w689 {
              selector: w689 -> [_ w705]
              tunnel: [i16 1 ("16bit integer") w705] -> w688
              frame 0 {
              }
              frame 1, Default {
              }
            }
            n403 = case shown="0" w687 {
              selector: w687 -> [_ w703]
              tunnel: [i16 1 ("16bit integer") w703] -> w686
              frame 0 {
              }
              frame 1, Default {
              }
            }
            n404 = Number To Decimal String(number=w686) -> (decimal integer string=w691:string)  [unwired: 1 in]
            n405 = Number To Decimal String(number=w688) -> (decimal integer string=w698:string)  [unwired: 1 in]
            n406 = Wait Until Next ms Multiple(millisecond multiple=u32 140) -> ()  [unwired: 1 out]
            n407 = Format Into String(format string="AXI1:SELSP 1:F1 %s:L1 %s:R1 1:AXI2:SELSP 2:F2 %s:L2 %s:R2 1", w698, w698, w691, w691) -> (resulting string=w697:string)  [unwired: 2 in, 1 out]
            n408 = call "D200_GPIB.vi"("GPIB\nAddress"=w696, "Write"=TRUE, "Read"=FALSE, "Characters to Write"=w697) -> ()  [unwired: 1 in, 3 out]
          }
        }
      }
    }
    frame 12 {
      n409 = stacked-sequence {
        frame #0 {
          n410 = local read "Radius"() -> (w727:i16)
          n411 = expression code="-2*x"(w727) -> (w726:i16)
          n412 = expression code="2*x"(w727) -> (w728:i16)
          n413 = local write "move x"(w726) -> ()
          n414 = local write "move y"(w728) -> ()
        }
        frame #1 {
          w746 = u16 1 ("L Speed")
          w737 = u16 1 ("L Speed")
          # "Move Y"
          # "Move X"
          n415 = local read "move x"() -> (w738:i16)
          n416 = local read "Motor GPIB"() -> (w731:u8)
          n417 = Greater?(x=w738, y=0) -> (0:w730:bool)
          n418 = Absolute Value(x=w738) -> (abs(x)=w735:i16)
          n419 = global write "X-Y Go(Global).vi" "x-axis"(w730) -> ()
          n420 = To Unsigned Long Integer(number=w735) -> (unsigned 32bit integer=w736:u32)
          n421 = call "Set_Parameter.vi"("Axis"=enum16{"X", "Y", "Z", "U", "V", "W"}."X", "Distance"=w736, "Rate"=u16 1, "L Speed"=w737, "F Speed"=w737, "GPIB_Addr"=w731) -> ()
          n422 = local read "move y"() -> (w744:i16)
          n423 = local read "Motor GPIB"() -> (w741:u8)
          n424 = Greater?(x=w744, y=0) -> (0:w729:bool)
          n425 = Absolute Value(x=w744) -> (abs(x)=w743:i16)
          n426 = global write "X-Y Go(Global).vi" "y-axis"(w729) -> ()
          n427 = To Unsigned Long Integer(number=w743) -> (unsigned 32bit integer=w745:u32)
          n428 = call "Set_Parameter.vi"("Axis"=enum16{"X", "Y", "Z", "U", "V", "W"}."Y", "Distance"=w745, "Rate"=u16 1, "L Speed"=w746, "F Speed"=w746, "GPIB_Addr"=w741) -> ()
        }
        frame #2 {
          n429 = local read "occurrence"() -> (w747:refnum<k4>)
          n430 = Set Occurrence(w747) -> ()
        }
        frame #3 {
          # "N=2*(2*pi*r)*90/(360*28)=pi*r/24"
          n431 = local read "Radius"() -> (w748:i16)
          n432 = formula code="N=pi*r/28;"("r"=w748) -> ("N"=w750:dbl)
          n433 = To Word Integer(number=w750) -> (16bit integer=w749:i16)
          n434 = local read "Motor GPIB"() -> (w752:u8)
          n435 = Number To Decimal String(number=w752) -> (decimal integer string=w751:string)  [unwired: 1 in]
          n436 = for {
            N: w749 -> [w756]
            tunnel: w751 -> [w758]
            i -> [w755]
            n437 = xnode "Formula"("i"=w755, "N"=w756) -> ("Result"=w754:dbl)  [unwired: 1 in, 1 out]
            n438 = xnode "Formula"("i"=w755, "N"=w756) -> ("Result"=w753:dbl)  [unwired: 1 in, 1 out]
            n439 = Wait Until Next ms Multiple(millisecond multiple=u32 140) -> ()  [unwired: 1 out]
            n440 = To Word Integer(number=w753) -> (16bit integer=w763:i16)
            n441 = To Word Integer(number=w754) -> (16bit integer=w770:i16)
            n442 = Number To Decimal String(number=w763) -> (decimal integer string=w762:string)  [unwired: 1 in]
            n443 = Number To Decimal String(number=w770) -> (decimal integer string=w764:string)  [unwired: 1 in]
            n444 = Format Into String(format string="AXI2:SELSP 1:F1 %s:L1 %s:R1 1", w762, w762) -> (resulting string=w765:string)  [unwired: 2 in, 1 out]
            n445 = Format Into String(format string="AXI1:SELSP 2:F2 %s:L2 %s:R2 1", w764, w764) -> (resulting string=w761:string)  [unwired: 2 in, 1 out]
            n446 = call "D200_GPIB.vi"("GPIB\nAddress"=w758, "Write"=TRUE, "Read"=FALSE, "Characters to Write"=w765) -> ()  [unwired: 1 in, 3 out]
            n447 = call "D200_GPIB.vi"("GPIB\nAddress"=w758, "Write"=TRUE, "Read"=FALSE, "Characters to Write"=w761) -> ()  [unwired: 1 in, 3 out]
          }
        }
      }
    }
  }
